vi "Fpga-Convert-TKeep-to-TKeep.vi"(11 "tkeep (MAC)":u8 format="%.0x") -> (3 "tkeep (MicroBlaze)":u8 format="%.0x")   [LabVIEW 2018]
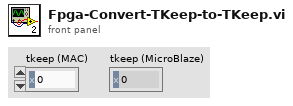
[diagram p1: front panel]
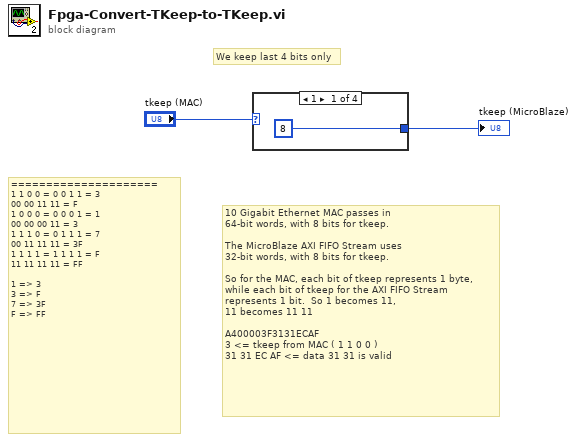
[diagram p0: block diagram]
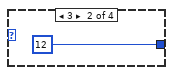
[diagram p2: hidden frame]
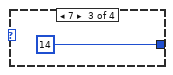
[diagram p3: hidden frame]
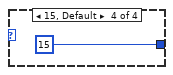
[diagram p4: hidden frame]
diagram:
  # "10 Gigabit Ethernet MAC passes in\n64-bit words, with 8 bits for tkeep.\n\nThe MicroBlaze AXI FIFO Stream uses\n32-bit words, with 8 bits for tkeep.\n\nSo for the MAC, each bit of tkeep represents 1 byte, \nwhile each bit of tkeep for the AXI FIFO Stream\nrepresents 1 bit.  So 1 becomes 11,\n11 becomes 11 11\n\nA400003F3131ECAF\n3 <= tkeep from MAC ( 1 1 0 0 )\n31 31 EC AF <= data 31 31 is valid"
  # "We keep last 4 bits only"
  # "=====================\n1 1 0 0 = 0 0 1 1 = 3\n00 00 11 11 = F\n1 0 0 0 = 0 0 0 1 = 1\n00 00 00 11 = 3\n1 1 1 0 = 0 1 1 1 = 7\n00 11 11 11 = 3F\n1 1 1 1 = 1 1 1 1 = F\n11 11 11 11 = FF\n\n1 => 3\n3 => F\n7 => 3F\nF => FF"
  n1 = case shown="1" "tkeep (MAC)" {
    tunnel: [u8 8 ("y") u8 12 ("y") u8 14 ("y") u8 15 ("y")] -> w1
    frame 1 {
    }
    frame 3 {
    }
    frame 7 {
    }
    frame 15, Default {
    }
  }
  "tkeep (MicroBlaze)" <- w1
